vi "convertPhysicalChannels.vi"(8 "error in (no error)":errorcluster, 10 "physicalChannels":string, 11 "DDSOutput in":refnum<class "DDSOutput.lvclass">) -> (0 "error out":errorcluster, 2 "physicalChannels":string[](array[string]), 3 "DDSOutput out":refnum<class "DDSOutput.lvclass">)   [LabVIEW 2009, in "Hardware.lvlib" / "Channels.lvlib" / "DDSOutput.lvclass"]
uses:
  DDSOutput.lvclass
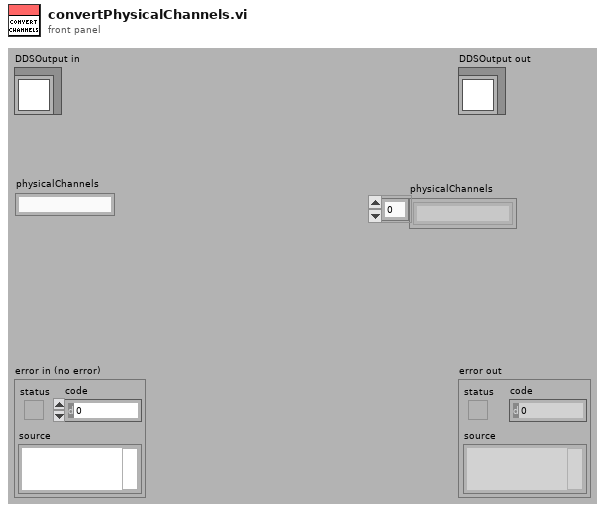
[diagram p1: front panel]
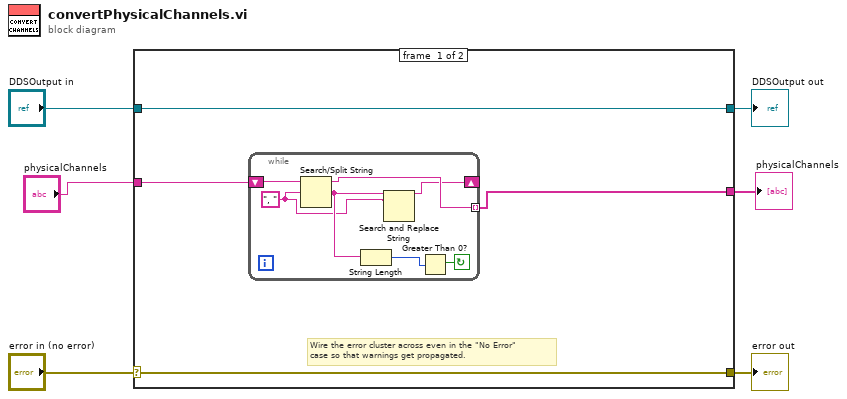
[diagram p0: block diagram]
diagram:
  n1 = case shown="No Error" "error in (no error)" {
    selector: "error in (no error)" -> [w9 w19]
    tunnel: [w9 w19] -> w5
    tunnel: [w10 w18] -> w3
    tunnel: "DDSOutput in" -> [w10 w18]
    tunnel: "physicalChannels" -> [w8 _]
    tunnel: [w7 _] -> w1
    frame #0 {
      # "Wire the error cluster across even in the \"No Error\"\ncase so that warnings get propagated."
      n2 = while {
        shift-right: [w13] -> _
        shift-left: w8 -> [w17]
        tunnel: [w16] -> w7 mode=indexing
        stop <- w11 continue-if-true
        w14 = ", "
        n3 = Search/Split String(string=w17, search string/char (-)=w14) -> (substring before match=w16:string, match + rest of string=w15:string)  [unwired: 1 in, 1 out]
        n4 = String Length(string=w15) -> (length=w12:i32)
        n5 = Search and Replace String(input string=w15, search string=w14) -> (result string=w13:string)  [unwired: 6 in, 3 out]
        n6 = Greater Than 0?(x=w12) -> (x > 0?=w11:bool)
      }
    }
    frame #1 {
    }
  }
  "error out" <- w5
  "DDSOutput out" <- w3
  "physicalChannels" <- w1
